vi "LCC Lookup Chan By Name.vi"(8 "error in (no error)":errorcluster caption="Fehler (Eingang, kein Fehler)", 11 "Channel Name":string) -> (0 "error out":errorcluster caption="Fehler (Ausgang)", 3 "Channel Handle":i64)   [LabVIEW 2021, in "labbCAN_Controller_API.lvlib"]
doc: "LCC_Func long LCC_CALL LCC_LookupChanByName(const char* pChannelName,\n dev_hdl* pChanHdl);"
uses:
  labbCAN_Controller_API.lvlib
  labbCAN_Controller_API.dll
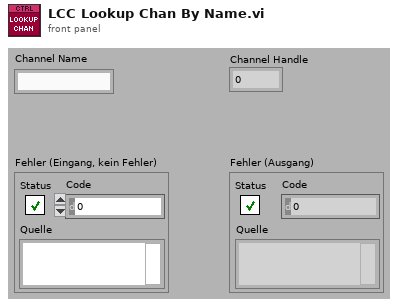
[diagram p1: front panel]
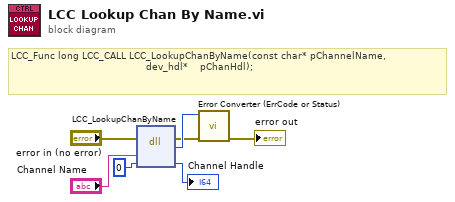
[diagram p0: block diagram]
diagram:
  # "LCC_Func long LCC_CALL LCC_LookupChanByName(const char* pChannelName,\n                                             dev_hdl*    pChanHdl);"
  n1 = dll-call lib="C:/Users/olaja/AppData/Local/CETONI_SDK/labbCAN_Controller_API.*" fn="LCC_LookupChanByName"(error in="error in (no error)", "pChannelName"="Channel Name", "pChanHdl"=i64 0) -> (error out=w2:errorcluster, "Rückgabetyp"=w3:i32, "pChanHdl"=→"Channel Handle":i64)  [unwired: 3 in, 1 out]
  n2 = call "Error Converter (ErrCode or Status).vi"("error in (no error)"=w2, "error code"=w3) -> ("error out"=→"error out":errorcluster)  [unwired: 9 in]
